vi "hmp4000 Read Current Output.vi"(8 "error in (no error)":errorcluster, 11 "VISA resource name":refnum<visa-resource-name>) -> (0 "error out":errorcluster, 2 "Current Value":dbl format="%.3f", 3 "VISA resource name out":refnum<visa-resource-name>)   [LabVIEW 2022 SP3]
doc: "This VI queries the measured Current value.\n\nAttribute:\nHMP4000_ATTR_MEASUREMENT_DC_CURRENT\n\nRemote-control command:\nMEASure:CURRent[:DC]?"
uses:
  Instance           1 35Saved   hmp4000 Read Current Output .vi
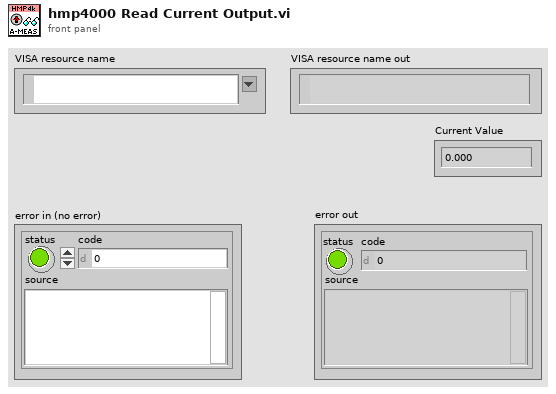
[diagram p1: front panel]
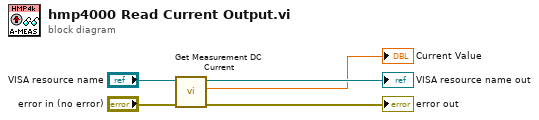
[diagram p0: block diagram]
diagram:
  n1 = call "Get Measurement DC Current"("error in (no error)"="error in (no error)", "instrument handle"="VISA resource name") -> ("error out"=→"error out":errorcluster, "Measurement DC Current"=→"Current Value":dbl, "instrument handle out"=→"VISA resource name out":refnum<visa-resource-name>)  [unwired: 7 in]
